vi "jt_keithley-2400_python.vi"(0 "Scan settings":T2={"J-V scan"=TRUE, "Start voltage (V)"=0.0, "End voltage (V)"=0.0, "Step voltage (V)"=1.4, "Scan both directions"=TRUE, "Inverted device structure"=FALSE, "Measurement delay (s)"=10.0, "Measurement speed"=0, "Scan rate (V/s)"=0.0, "Stabilisation time (s)"=0.0, "Stabilisation mode"=0, "Stabilisation value (V or A) "=1.0, "Illumination"=0, "Stabilisation in the dark?"=FALSE, "Repeat light scans"=FALSE, "No. of repeat scans"=0.0, "Only repeat for best pixel"=1, "J-t scan"=FALSE, "J-t best pixel only"=7, "J-t start voltage (V)"=0.0, "J-t end voltage (V)"=1.4, "J-t step voltage (V)"=0.01, "Step time (s)"=0.7, "J-t scan both directions"=TRUE, "J-t inverted device structure"=FALSE, "Settling delay (s)"=0.0, "J-t measurement speed"=0, "J-t illumination"=2, "Max. power stabilisation"=FALSE, "Max power best pixel only"=1, "Max. power point tracker"=FALSE, "Vmp from J-V scan"=FALSE, "Max P stab. Specific voltage"=FALSE, "Vmp (V)"=1.0, "Stabilisation time step (s)"=1.0, "Total stabilisation time (s)"=100.0} {"Settling delay (s)" min=0.0; "J-t illumination" items=["Light only", "Dark only", "Light then dark", "Dark then light"]; "Measurement speed" items=["Fast", "Normal", "High accuracy"]; "Illumination" items=["Light only", "Dark only", "Light then dark", "Dark then light"]; "Only repeat for best pixel" items=["only for best pixel", "for best 2 pixels", "for best 3 pixels", "for best 4 pixels", "for best 5 pixels", "for best 6 pixels", "for best 7 pixels", "for all pixels"]; "No. of repeat scans" min=1.0 step=1.0; "Max power best pixel only" items=["only the best pixel", "the best 2 pixels", "the best 3 pixels", "the best 4 pixels", "the best 5 pixels", "the best 6 pixels", "the best 7 pixels", "all pixels"]; "J-t best pixel only" items=["only the best pixel", "the best 2 pixels", "the best 3 pixels", "the best 4 pixels", "the best 5 pixels", "the best 6 pixels", "the best 7 pixels", "all pixels"]; "J-t measurement speed" items=["Fast", "Normal", "High Accuracy"]; "Stabilisation mode" items=["V", "I"]; "Measurement delay (s)" min=0.01}, 1 "file name":string, 2 "folder path":string, 5 "Cell details cluster":T1={"Cell Position"=16, "Cell Label"="", "Pixel to measure"=0, "Area (cm^2)"=0.126, "Variable"="", "Variable value"="", "Scan settings in queue"=0, "Light or dark"="", "Measurement Type"=""} {"Pixel to measure" items=["All", "1", "2", "3", "4", "5", "6", "7", "8"]}, 11 "error in (no error)":errorcluster, 12 "illumination intensity (suns equiv.)":string) -> (15 "error out":errorcluster)   [LabVIEW 2016]
uses:
  TypeDefs/scan_settings.ctl
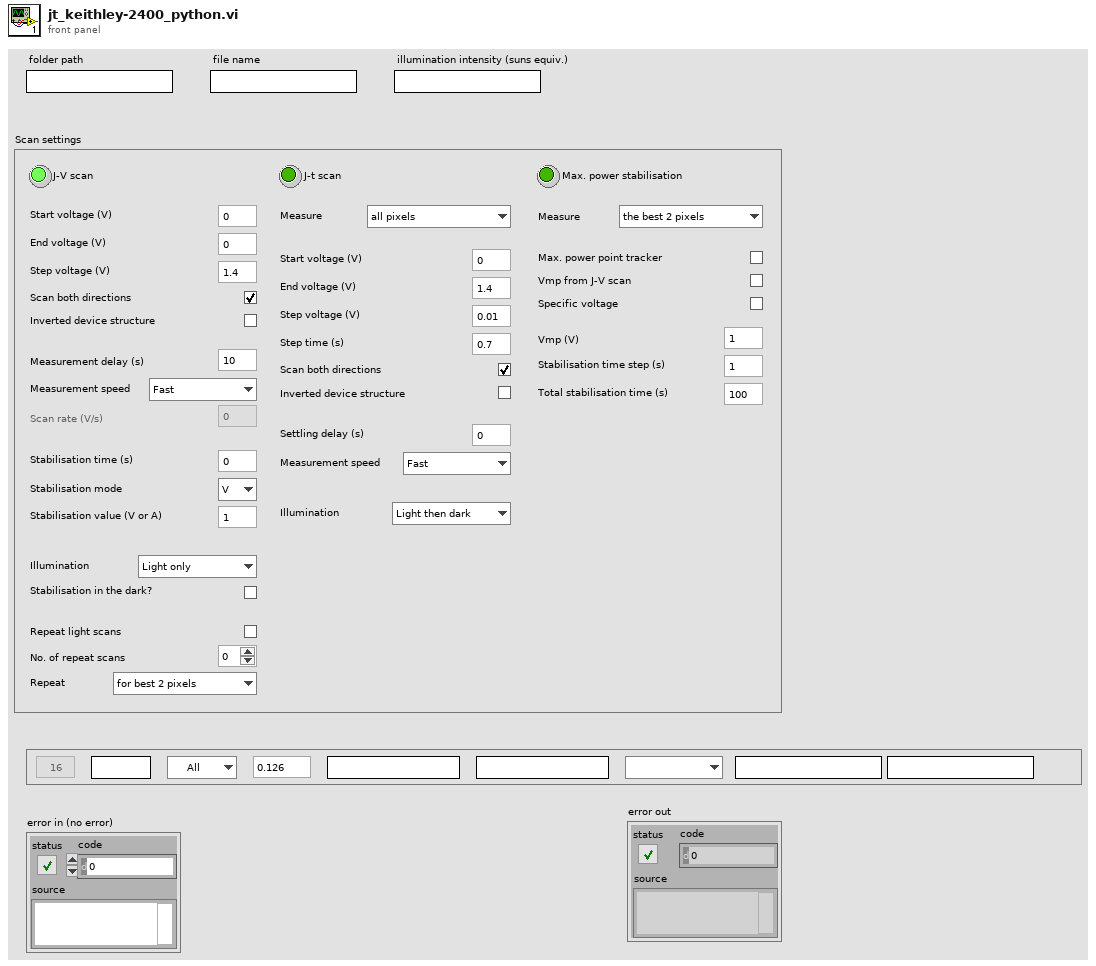
[diagram p1: front panel]
types:
  T1 = cluster{"Cell Position":i32, "Cell Label":string, "Pixel to measure":u16, "Area (cm^2)":dbl, "Variable":string, "Variable value":string, "Scan settings in queue":u16, "Light or dark":string, "Measurement Type":string}
  T2 = typedef "scan_settings.ctl" = cluster{"J-V scan":bool, "Start voltage (V)":dbl, "End voltage (V)":dbl, "Step voltage (V)":dbl, "Scan both directions":bool, "Inverted device structure":bool, "Measurement delay (s)":dbl, "Measurement speed":u8, "Scan rate (V/s)":dbl, "Stabilisation time (s)":dbl, "Stabilisation mode":u16, "Stabilisation value (V or A) ":dbl, "Illumination":u16, "Stabilisation in the dark?":bool, "Repeat light scans":bool, "No. of repeat scans":dbl, "Only repeat for best pixel":u16, "J-t scan":bool, "J-t best pixel only":u16, "J-t start voltage (V)":dbl, "J-t end voltage (V)":dbl, "J-t step voltage (V)":dbl, "Step time (s)":dbl, "J-t scan both directions":bool, "J-t inverted device structure":bool, "Settling delay (s)":dbl, "J-t measurement speed":u16, "J-t illumination":u16, "Max. power stabilisation":bool, "Max power best pixel only":u16, "Max. power point tracker":bool, "Vmp from J-V scan":bool, "Max P stab. Specific voltage":bool, "Vmp (V)":dbl, "Stabilisation time step (s)":dbl, "Total stabilisation time (s)":dbl}
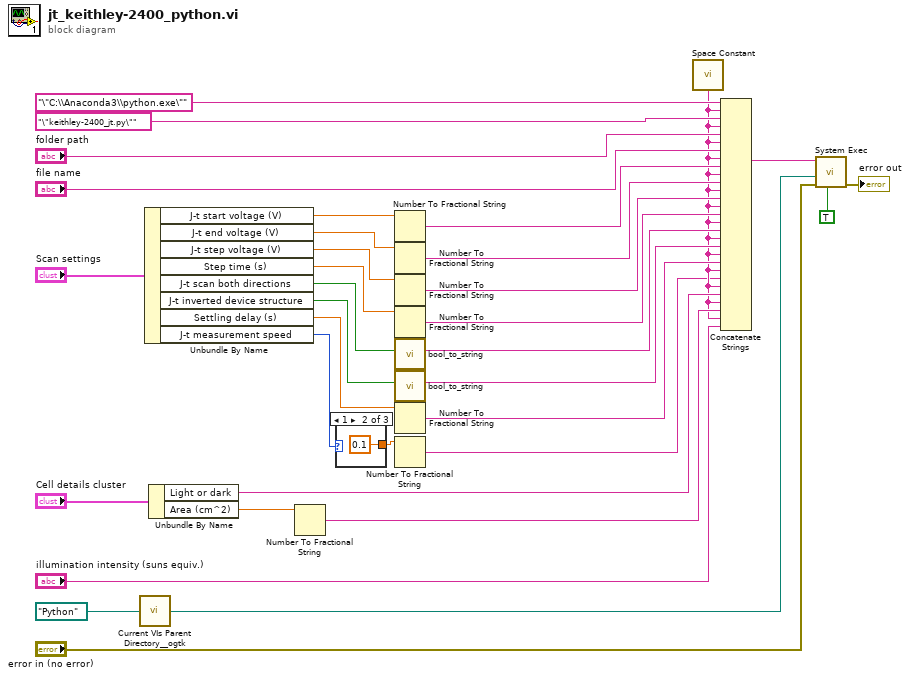
[diagram p0: block diagram]
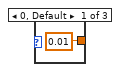
[diagram p2: hidden frame]
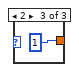
[diagram p3: hidden frame]
diagram:
  n1 = call <userlib>:"Current VIs Parent Directory__ogtk.vi"("Relative path (.)"=path "Python") -> ("Parent Directory (+ Relative)"=w2:path)  [unwired: 4 in]
  n2 = Unbundle By Name("Scan settings") -> ("J-t start voltage (V)"=w25:dbl, "J-t end voltage (V)"=w24:dbl, "J-t step voltage (V)"=w23:dbl, "Step time (s)"=w22:dbl, "J-t scan both directions"=w21:bool, "J-t inverted device structure"=w20:bool, "Settling delay (s)"=w19:dbl, "J-t measurement speed"=w17:u16)
  n3 = Unbundle By Name("Cell details cluster") -> ("Light or dark"=w7:string, "Area (cm^2)"=w8:dbl)
  n4 = Number To Fractional String(number=w8) -> (F-format string=w6:string)  [unwired: 3 in]
  n5 = case shown="1" w17 {
    tunnel: [0.01 0.1 1] -> w18
    frame 0, Default {
    }
    frame 1 {
    }
    frame 2 {
    }
  }
  n6 = Number To Fractional String(number=w25) -> (F-format string=w15:string)  [unwired: 3 in]
  n7 = Number To Fractional String(number=w24) -> (F-format string=w14:string)  [unwired: 3 in]
  n8 = Number To Fractional String(number=w23) -> (F-format string=w13:string)  [unwired: 3 in]
  n9 = Number To Fractional String(number=w22) -> (F-format string=w12:string)  [unwired: 3 in]
  n10 = call "bool_to_string.vi"("Boolean"=w21) -> ("String"=w11:string)  [unwired: 10 in]
  n11 = call "bool_to_string.vi"("Boolean"=w20) -> ("String"=w10:string)  [unwired: 10 in]
  n12 = Number To Fractional String(number=w19) -> (F-format string=w9:string)  [unwired: 3 in]
  n13 = Number To Fractional String(number=w18) -> (F-format string=w4:string)  [unwired: 3 in]
  n14 = call <vilib>:"Space Constant.vi"() -> ("String"=w5:string)
  n15 = Concatenate Strings("\"C:\\Anaconda3\\python.exe\"" ("standard input"), w5, "\"keithley-2400_jt.py\"" ("standard input"), w5, "folder path", w5, "file name", w5, w15, w5, w14, w5, w13, w5, w12, w5, w11, w5, w10, w5, w9, w5, w4, w5, w7, w5, w6, w5, "illumination intensity (suns equiv.)") -> (w32:string)
  n16 = call <vilib>:"System Exec.vi"("run minimized? (F)"=TRUE, "error in (no error)"="error in (no error)", "working directory"=w2, "command line"=w32) -> ("error out"=→"error out":errorcluster)  [unwired: 4 in, 3 out]
